vi "PanelWizard_ConfigurePanelWizardDialog.vi"(11 "Display State":T2={"DisplayStyle"=enum."3D Style", "LaunchType"=enum."LaunchHDV", "UserVIPath"=path "", "Button Text"="", "UseDefaultButtonText?"=FALSE, "Run User VI?"=TRUE, "CommandLine"="", "StandardInput"="", "Working Directory"=path ""} caption="State") -> (1 "Updated?":bool, 3 "Display State Out":T2={"DisplayStyle"=enum."3D Style", "LaunchType"=enum."LaunchHDV", "UserVIPath"=path "", "Button Text"="", "UseDefaultButtonText?"=FALSE, "Run User VI?"=TRUE, "CommandLine"="", "StandardInput"="", "Working Directory"=path ""} caption="State")   [LabVIEW 2012, in "PanelWizard.xctl"]
doc: "Use this template to create a dialog box with event handling."
uses:
  PanelWizard.xctl
  PanelWizard_State.ctl
  PanelWizard_DisplayType.ctl
  PanelWizard_LaunchOptions.ctl
panel:
  in  "Display Style":T1
  in  "Use Custom Label?":bool
  in  "Button Text":string
  in  "Action Configuration Pages":T4(tab)=enum."LaunchUserVI"
  in  "Run VI?":bool=TRUE
  in  "Path":path
  in  "Working Directory":path
  in  "Standard Input":string
  in  "Command Line":string
  in  "Choose an action":i32(listbox)
  in  "Cancel":bool
  in  "OK":bool
  # "Launch the Historical Data viewer"
  # "Launch System Manager"
  # "Launch a user vi"
  # "Run command line"
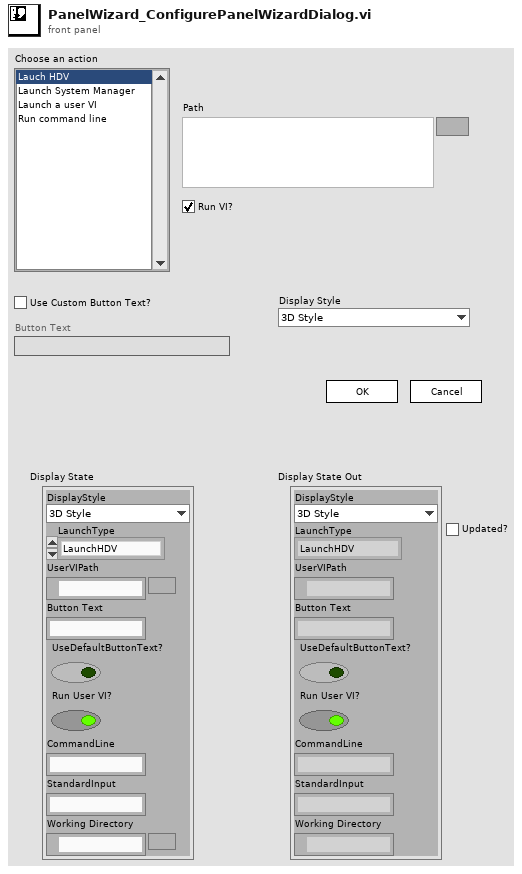
[diagram p1: front panel]
types:
  T1 = typedef "PanelWizard.xctl/PanelWizard_DisplayType.ctl" = enum16{"3D Style", "LabVIEW Classic Style", "System Style"}
  T2 = typedef "PanelWizard.xctl/PanelWizard_State.ctl" = cluster{"DisplayStyle":T1, "LaunchType":T3, "UserVIPath":path, "Button Text":string, "UseDefaultButtonText?":bool, "Run User VI?":bool, "CommandLine":string, "StandardInput":string, "Working Directory":path}
  T3 = typedef "PanelWizard.xctl/PanelWizard_LaunchOptions.ctl" = enum16{"LaunchHDV", "LaunchSVMonitor", "LaunchUserVI", "Run command line"}
  T4 = enum32{"LaunchHDV", "LaunchSVMonitor", "LaunchUserVI", "Run command line"}
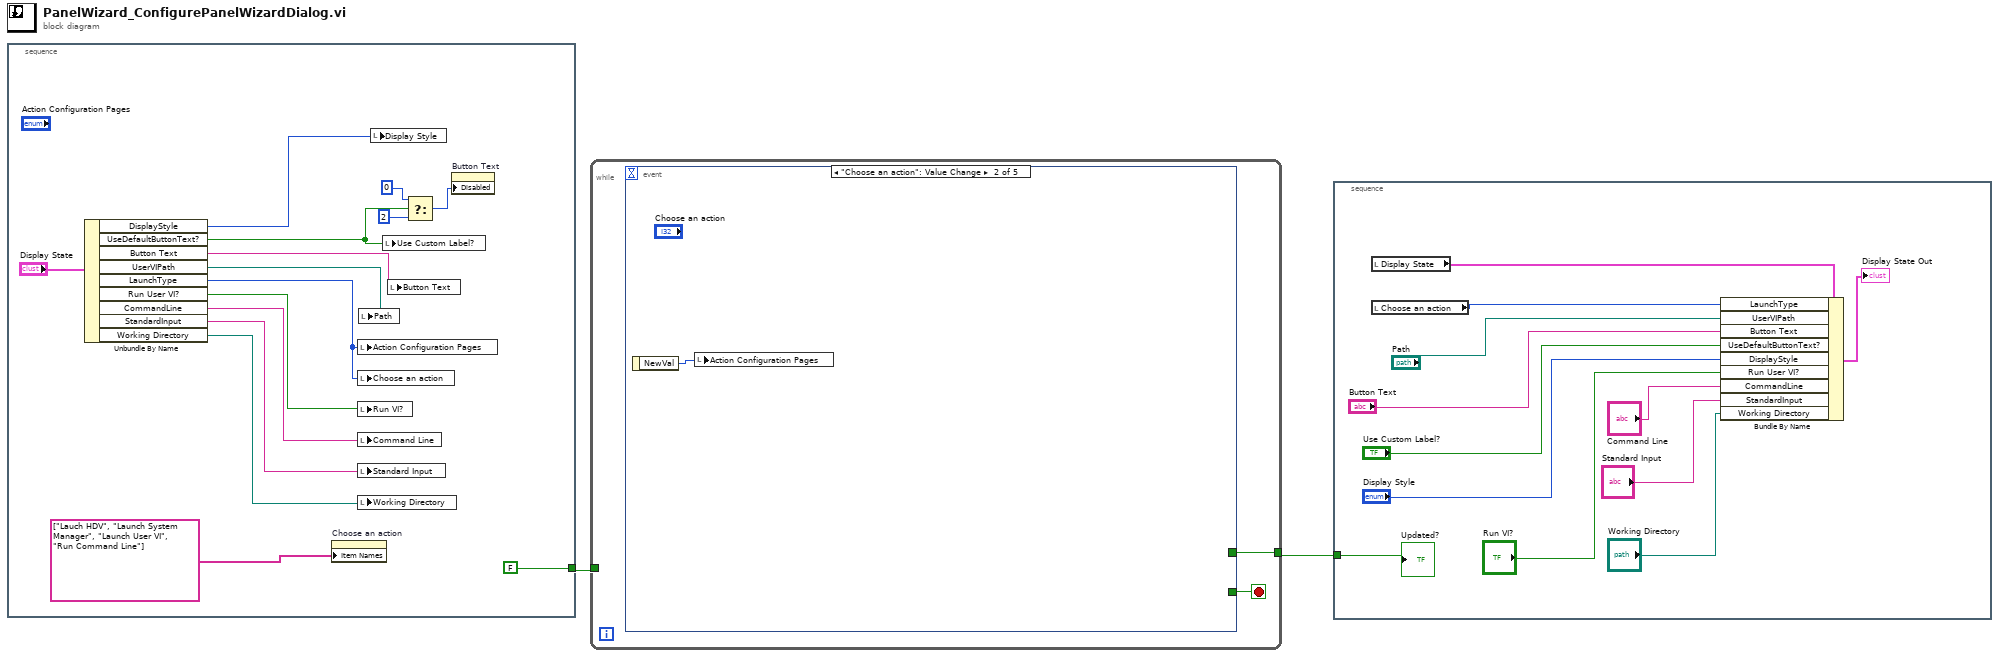
[diagram p0: block diagram]
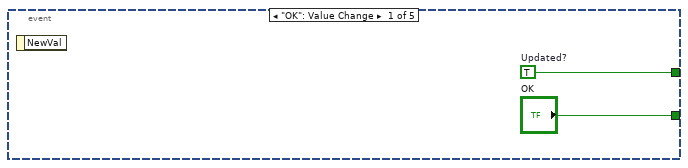
[diagram p2: hidden frame]
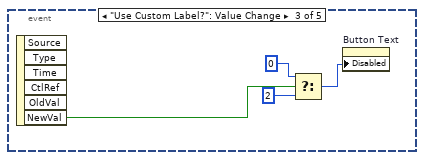
[diagram p3: hidden frame]
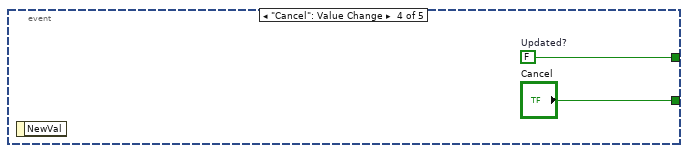
[diagram p4: hidden frame]
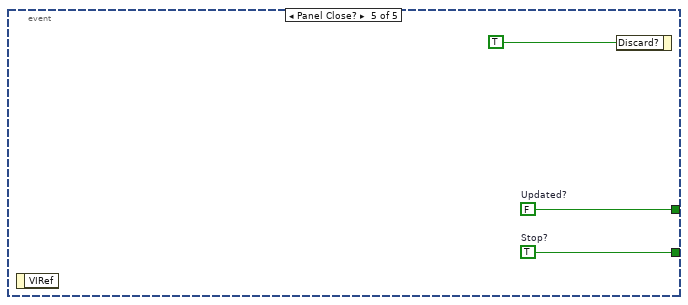
[diagram p5: hidden frame]
diagram:
  n1 = stacked-sequence {
    tunnel: [FALSE ("NewVal")] -> w1
    frame #0 {
      n2 = Unbundle By Name("Display State") -> ("DisplayStyle"=w7:T1, "UseDefaultButtonText?"=w11:bool, "Button Text"=w12:string, "UserVIPath"=w13:path, "LaunchType"=w14:T3, "Run User VI?"=w6:bool, "CommandLine"=w5:string, "StandardInput"=w4:string, "Working Directory"=w3:path)
      n3 = property on="Choose an action" class="LstBox (strict)"("Item Names"=string[] ["Lauch HDV", "Launch System Manager", "Launch User VI", "Run Command Line"]) -> ()  [unwired: 2 in, 2 out]
      n4 = local write "Action Configuration Pages"(w14) -> ()
      n5 = local write "Choose an action"(w14) -> ()
      n6 = local write "Run VI?"(w6) -> ()
      n7 = local write "Command Line"(w5) -> ()
      n8 = local write "Standard Input"(w4) -> ()
      n9 = local write "Working Directory"(w3) -> ()
      n10 = local write "Path"(w13) -> ()
      n11 = local write "Display Style"(w7) -> ()
      n12 = local write "Use Custom Label?"(w11) -> ()
      n13 = local write "Button Text"(w12) -> ()
      n14 = Select(t=u8 0 ("Disabled"), s=w11, f=u8 2 ("Disabled")) -> (s? t:f=w8:u8)
      n15 = property on="Button Text" class="Str"("Disabled"=w8) -> ()  [unwired: 2 in, 2 out]
    }
  }
  n16 = while {
    tunnel: [w18] -> w2
    tunnel: w1 -> [_]
    stop <- w19 stop-if-true
    n17 = event shown="[1] \"Choose an action\": Value Change" {
      selector: _ -> [_ _ _ _ _]
      dyn-events: _ -> [_ _ _ _ _]
      timeout: _ -> [_ _ _ _ _]
      tunnel: ["OK" _ _ "Cancel" w30] -> w19
      tunnel: [w21 _ _ w28 w29] -> w18
      event "OK": Value Change {
        w21 = TRUE  # Updated?
        n18 = event-data() -> ()  [unwired: 1 in, 1 out]
      }
      event "Choose an action": Value Change {
        n19 = event-data() -> ("NewVal"=w22:i32)  [unwired: 1 in]
        n20 = local write "Action Configuration Pages"(w22) -> ()
      }
      event "Use Custom Label?": Value Change {
        n21 = event-data() -> ("NewVal"=w23:bool)  [unwired: 1 in, 5 out]
        n22 = Select(t=u8 0 ("Disabled"), s=w23, f=u8 2 ("Disabled")) -> (s? t:f=w24:u8)
        n23 = property on="Button Text" class="Str"("Disabled"=w24) -> ()  [unwired: 2 in, 2 out]
      }
      event "Cancel": Value Change {
        w28 = FALSE  # Updated?
        n24 = event-data() -> ()  [unwired: 1 in, 1 out]
      }
      event Panel Close? {
        w29 = FALSE  # Updated?
        w30 = TRUE  # Stop?
        n25 = event-data() -> ()  [unwired: 1 in, 1 out]
        n26 = event-data("Discard?"=TRUE) -> ()  [unwired: 1 in, 1 out]
      }
    }
  }
  n27 = stacked-sequence {
    tunnel: w2 -> [w43]
    frame #0 {
      n28 = local read "Display State"() -> (w42:T2)
      n29 = local read "Choose an action"() -> (w41:i32)
      n30 = Bundle By Name(cluster=w42, "LaunchType"=w41, "UserVIPath"="Path", "Button Text"="Button Text", "UseDefaultButtonText?"="Use Custom Label?", "DisplayStyle"="Display Style", "Run User VI?"="Run VI?", "CommandLine"="Command Line", "StandardInput"="Standard Input", "Working Directory"="Working Directory") -> (→"Display State Out":T2)
      "Updated?" <- w43
    }
  }
